vi "Process Directors.vi"(8 "error in (no error)":errorcluster, 9 "Results Notifier":refnum<notifier>, 10 "Wait Time":u32 caption="ms" step=1, 11 "InteractionProcessor in":refnum<class "InteractionProcessor.lvclass">) -> (0 "error out":errorcluster, 3 "InteractionProcessor out":refnum<class "InteractionProcessor.lvclass">)   [LabVIEW 2023, in "HAF.lvlib" / "InteractionProcessor.lvclass"]
doc: "Processes all Command Directors until they complete. This member will respond to events to Pause, Resume and Stop. Results will be notified on the Notification Queue."
uses:
  InteractionProcessor.lvclass
  ReadCommand/ReadCommand.lvclass
  Global Resources.vi
  HAF.lvlib
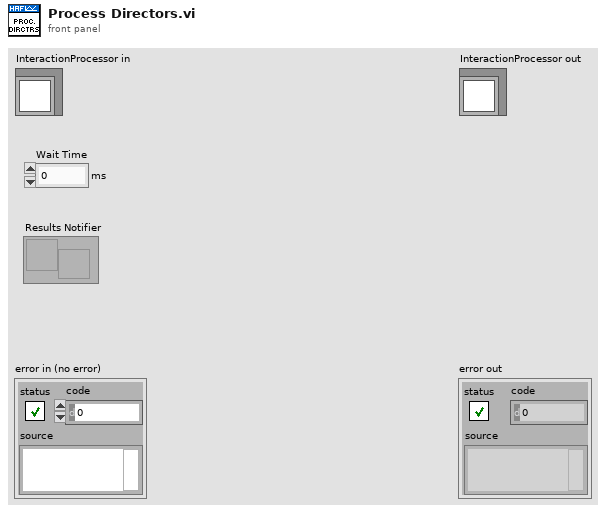
[diagram p1: front panel]
types:
  T1 = typedef "HAF.lvlib/All Message Queues.ctl" = cluster{"Internal":refnum<queue>, "Notifications":refnum<queue>}
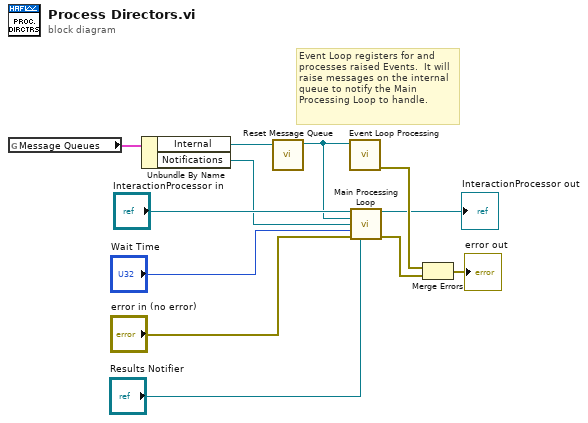
[diagram p0: block diagram]
diagram:
  # "Event Loop registers for and \nprocesses raised Events.  It will\nraise messages on the internal\nqueue to notify the Main \nProcessing Loop to handle."
  n1 = global read "Global Resources.vi" "Message Queues"() -> (w12:T1)
  n2 = Unbundle By Name(w12) -> ("Internal"=w11:refnum<queue>, "Notifications"=w4:refnum<queue>)
  n3 = call "Reset Message Queue.vi"("Message Queue In"=w11) -> ("Message Queue Out"=w3:refnum<queue>)  [unwired: 9 in, 1 out]
  n4 = call "Event Loop Processing.vi"("Message Queue In"=w3) -> ("error out"=w6:errorcluster)  [unwired: 10 in]
  n5 = call "Main Processing Loop.vi"("InteractionProcessor in"="InteractionProcessor in", "Internal Message Queue"=w3, "Notification Message Queue"=w4, "Wait Time"="Wait Time", "error in (no error)"="error in (no error)", "Results Notifier"="Results Notifier") -> ("InteractionProcessor out"=→"InteractionProcessor out":refnum<class "InteractionProcessor.lvclass">, "error out"=w7:errorcluster)  [unwired: 8 in]
  n6 = Merge Errors(w6, w7) -> (→"error out":errorcluster)
